vi "Read Calibration Factors.vi"(8 "error in (no error)":errorcluster, 11 "VGC in":refnum<class "PL Inficon VGC.lvclass">) -> (0 "error out":errorcluster, 2 "calibration factors":dbl[](array[numeric]), 3 "VGC out":refnum<class "PL Inficon VGC.lvclass">)   [LabVIEW 2015, in "PL Inficon VGC.lvclass"]
doc: "Reads calibration factors."
uses:
  PL Inficon VGC.lvclass
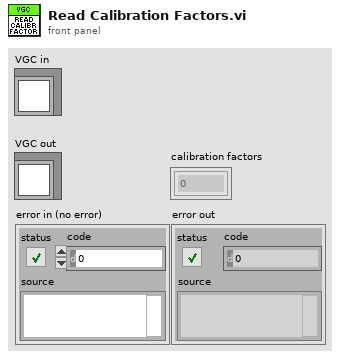
[diagram p1: front panel]
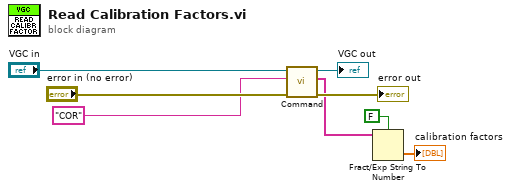
[diagram p0: block diagram]
diagram:
  n1 = call "Command.vi"("error in (no error)"="error in (no error)", "command"="COR" ("format string"), "VGC in"="VGC in") -> ("error out"=→"error out":errorcluster, "response data"=w2:string[], "VGC out"=→"VGC out":refnum<class "PL Inficon VGC.lvclass">)  [unwired: 6 in]
  n2 = Fract/Exp String To Number(use system decimal point (T)=FALSE, string=w2) -> (number=→"calibration factors":dbl[])  [unwired: 2 in, 1 out]
